vi "TW Recursive SubVIs.vi"(8 "error in (no error)":errorcluster, 9 "Constant references in in":refnum<vi>[](array[refnum]), 10 "SubVI references in in":refnum<vi>[](array[refnum]), 11 "Diagrams in":refnum<vi>[](array[refnum])) -> (0 "error out":errorcluster, 1 "Constant references out":refnum<vi>[](array[refnum]), 2 "SubVI references out":refnum<vi>[](array[refnum]))   [LabVIEW 2021]
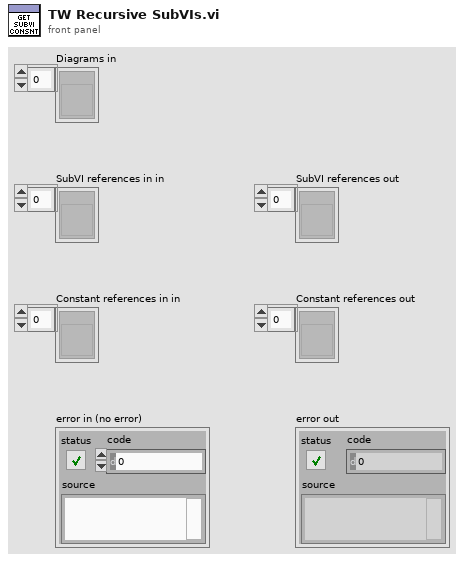
[diagram p1: front panel]
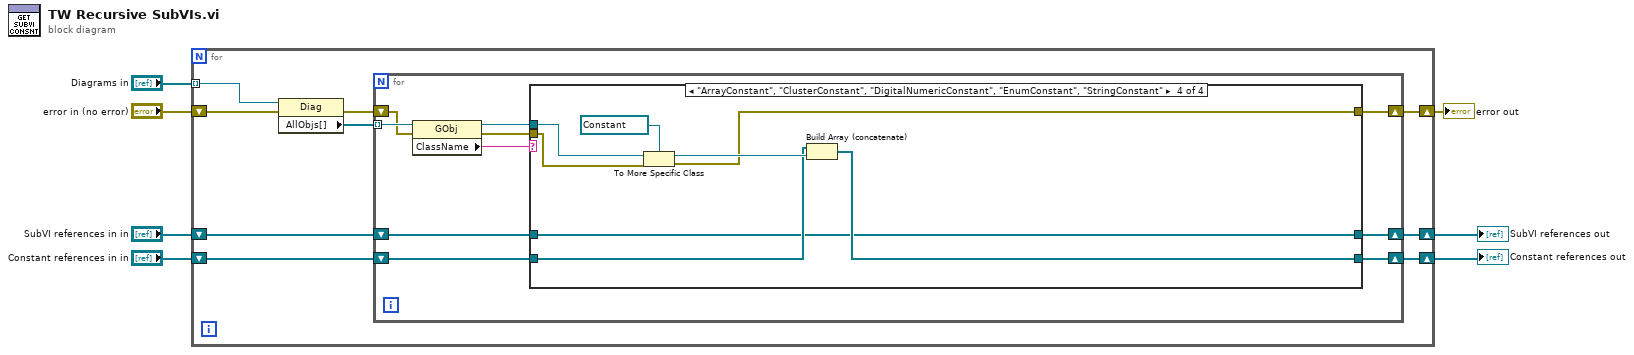
[diagram p0: block diagram]
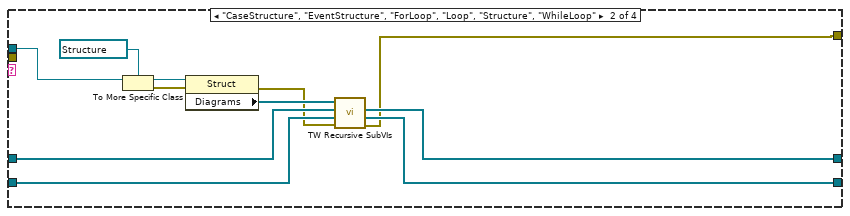
[diagram p3: hidden frame]
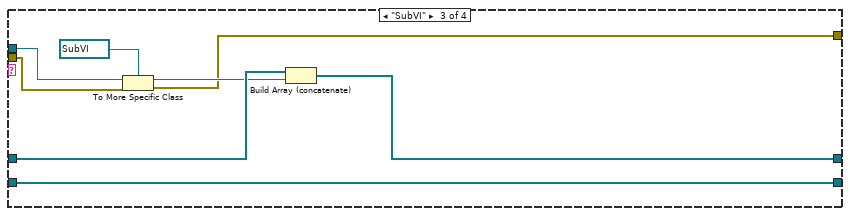
[diagram p4: hidden frame]
diagram:
  n1 = for {
    tunnel: "Diagrams in" -> [w9] mode=indexing
    shift-right: [w14] -> w1
    shift-left: "SubVI references in in" -> [w15]
    shift-right: [w12] -> w4
    shift-left: "Constant references in in" -> [w13]
    shift-right: [w8] -> w2
    shift-left: "error in (no error)" -> [w11]
    n2 = property class="Diag"(reference=w9, error in=w11) -> (error out=w10:errorcluster, "AllObjs[]"=w16:refnum<vi>[])  [unwired: 1 out]
    n3 = for {
      tunnel: w16 -> [w26] mode=indexing
      shift-right: [w22] -> w14
      shift-left: w15 -> [w23]
      shift-right: [w20] -> w12
      shift-left: w13 -> [w21]
      shift-right: [w17] -> w8
      shift-left: w10 -> [w19]
      n4 = property class="GObj"(reference=w26, error in=w19) -> (reference out=w25:refnum<vi>, error out=w18:errorcluster, "ClassName"=w24:string)
      n5 = case shown="\"ArrayConstant\", \"ClusterConstant\", \"DigitalNumericConstant\", \"EnumConstant\", \"StringConstant\"" w24 {
        tunnel: w25 -> [_ w37 w47 w55]
        tunnel: w23 -> [w29 w35 w45 w49]
        tunnel: [w29 w34 w43 w49] -> w22
        tunnel: w21 -> [w28 w33 w46 w51]
        tunnel: [w28 w32 w46 w50] -> w20
        tunnel: w18 -> [w27 _ w42 w53]
        tunnel: [w27 w30 w41 w52] -> w17
        frame "False", Default {
        }
        frame "CaseStructure", "EventStructure", "ForLoop", "Loop", "Structure", "WhileLoop" {
          n6 = To More Specific Class(target class=refnum<vi> refnum ("reference"), reference=w37) -> (specific class reference=w39:refnum<vi>, error out=w40:errorcluster)  [unwired: 1 in]
          n7 = property class="Struct"(reference=w39, error in=w40) -> (error out=w31:errorcluster, "Diagrams"=w36:refnum<vi>[])  [unwired: 1 out]
          n8 = call "TW Recursive SubVIs.vi"("error in (no error)"=w31, "Constant references in in"=w33, "SubVI references in in"=w35, "Diagrams in"=w36) -> ("error out"=w30:errorcluster, "Constant references out"=w32:refnum<vi>[], "SubVI references out"=w34:refnum<vi>[])  [unwired: 5 in]
        }
        frame "SubVI" {
          n9 = To More Specific Class(target class=refnum<vi> refnum ("reference"), reference=w47, error in=w42) -> (specific class reference=w44:refnum<vi>, error out=w41:errorcluster)
          n10 = Build Array (concatenate)(w45, w44) -> (w43:refnum<vi>[])
        }
        frame "ArrayConstant", "ClusterConstant", "DigitalNumericConstant", "EnumConstant", "StringConstant" {
          n11 = To More Specific Class(target class=refnum<vi> refnum ("reference"), reference=w55, error in=w53) -> (specific class reference=w54:refnum<vi>, error out=w52:errorcluster)
          n12 = Build Array (concatenate)(w51, w54) -> (w50:refnum<vi>[])
        }
      }
    }
  }
  "Constant references out" <- w4
  "SubVI references out" <- w1
  "error out" <- w2
